vi "Write GPIO wrackpos2023.vi"(0 "Lines":tag="Dev1/port0/line0:7,Dev1/port1/line0:7,Dev1/port2/line0:7", 1 "EFC":bool, 2 "Position":i8=1 min=1 max=32, 3 "Rack Pos":i8, 6 "VTEST EN":bool=TRUE, 7 "RF EN":bool) -> ()   [LabVIEW 2023]
doc: "I. Description:\nThis example demonstrates how to write values to a digital output channel.\n\nII. Instructions for Running:\n1. Select the digital lines on the DAQ device to be written.\n2. Select a value to write.\nNote: The array control is sized for 8 lines, if using a different amount of lines, change the number of elements in the array to equal the number of lines chosen.\n\nIII. Block Diagram Steps:\n1. Create a Digital Output channel. Use one channel for all lines. You can alternatively use one channel for each line, but then use a different polymorphic version of the DAQmx Write VI.\n2. Call the Start VI to start the task.\n3. Write the digital Boolean array data in a loop until the user hits the stop button or an error occurs. This write VI writes a single sample of digital data on demand, so no timeout is necessary.\n4. Call the Clear Task VI to clear the Task.\n5. Use the popup dialog box to display an error or warning if any.\n\nIV. I/O Connections Overview:\nMake sure your signal output terminals match the Lines I/O Control. In this case wire the item to receive the signal to the first eight digital lines on your DAQ Device."
uses:
  <vilib>/Utility/error.llb/DialogType.ctl
  <vilib>/DAQmx/write.llb/DAQmx Write (Digital 1D Bool 1Chan 1Samp).vi
  <vilib>/DAQmx/create/channels.llb/DAQmx Create Channel (DO-Digital Output).vi
  <vilib>/DAQmx/miscellaneous.llb/DAQmx Fill In Error Info.vi
panel:
  # "For instructions, select Help>>Show Context Help"
  # "Channel Parameters"
  # "*The number of lines in the list must\nmatch the number of elements in\nthe array."
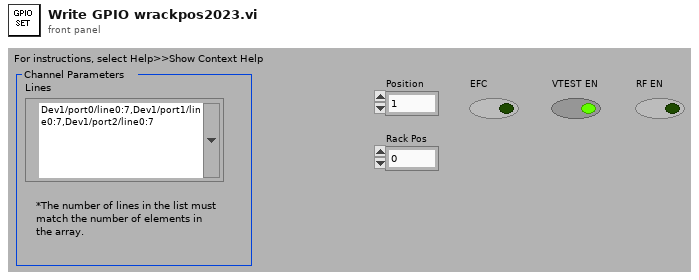
[diagram p1: front panel]
types:
  T1 = typedef "DialogType.ctl" = u16
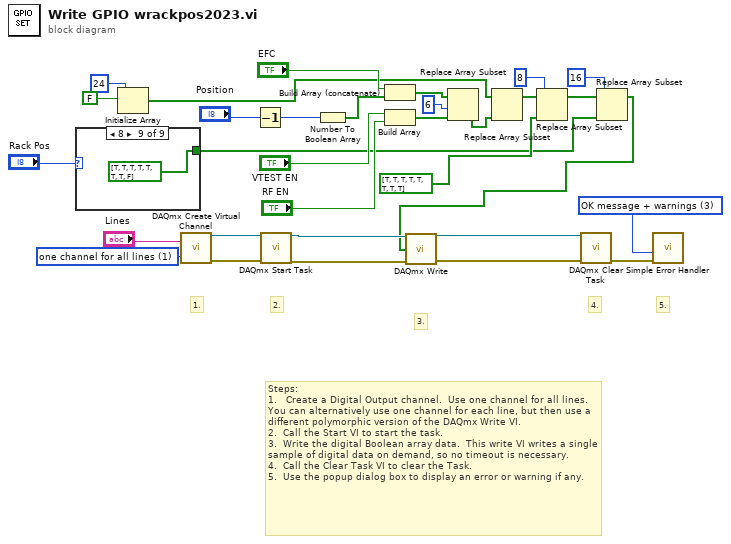
[diagram p0: block diagram]
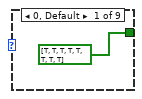
[diagram p2: hidden frame]
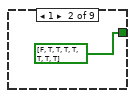
[diagram p3: hidden frame]
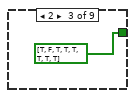
[diagram p4: hidden frame]
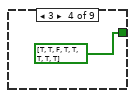
[diagram p5: hidden frame]
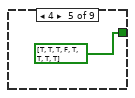
[diagram p6: hidden frame]
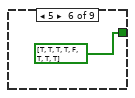
[diagram p7: hidden frame]
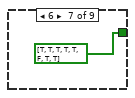
[diagram p8: hidden frame]
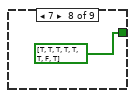
[diagram p9: hidden frame]
diagram:
  w26 = 1 items=["one channel for each line", "one channel for all lines"] ("line grouping")
  w27 = T1 3 items=["no dialog", "OK message", "continue or stop message", "OK message + warnings", "continue/stop + warnings"] ("type of dialog (OK msg:1)")
  # "3."
  # "5."
  # "Steps: \n1.   Create a Digital Output channel.  Use one channel for all lines.  You can alternatively use one channel for each line, but then use a different polymorphic version of the DAQmx Write VI.\n2.  Call the Start VI to start the task.\n3.  Write the digital Boolean array data.  This write VI writes a single sample of digital data on demand, so no timeout is necessary.\n4.  Call the Clear Task VI to clear the Task.\n5.  Use the popup dialog box to display an error or warning if any."
  # "4."
  # "2."
  # "1."
  n1 = case shown="8" "Rack Pos" {
    tunnel: [bool[] [TRUE, TRUE, TRUE, TRUE, TRUE, TRUE, TRUE, TRUE] bool[] [FALSE, TRUE, TRUE, TRUE, TRUE, TRUE, TRUE, TRUE] bool[] [TRUE, FALSE, TRUE, TRUE, TRUE, TRUE, TRUE, TRUE] bool[] [TRUE, TRUE, FALSE, TRUE, TRUE, TRUE, TRUE, TRUE] bool[] [TRUE, TRUE, TRUE, FALSE, TRUE, TRUE, TRUE, TRUE] bool[] [TRUE, TRUE, TRUE, TRUE, FALSE, TRUE, TRUE, TRUE] bool[] [TRUE, TRUE, TRUE, TRUE, TRUE, FALSE, TRUE, TRUE] bool[] [TRUE, TRUE, TRUE, TRUE, TRUE, TRUE, FALSE, TRUE] bool[] [TRUE, TRUE, TRUE, TRUE, TRUE, TRUE, TRUE, FALSE]] -> w1
    frame 0, Default {
    }
    frame 1 {
    }
    frame 2 {
    }
    frame 3 {
    }
    frame 4 {
    }
    frame 5 {
    }
    frame 6 {
    }
    frame 7 {
    }
    frame 8 {
    }
  }
  n2 = Initialize Array(FALSE, 24 ("dimension size")) -> (w10:bool[])
  n3 = call-poly <vilib>:"DAQmx Create Virtual Channel.vi"("lines"="Lines", "line grouping"=w26) -> ("task out"=w30:refnum<k21>, "error out"=w29:errorcluster)  [unwired: 12 in]
  n4 = Decrement(x="Position") -> (x-1=w14:i8)
  n5 = call <vilib>:"DAQmx Start Task.vi"("task/channels in"=w30, "error in"=w29) -> ("task out"=w25:refnum<k21>, "error out"=w24:errorcluster)  [unwired: 12 in]
  n6 = Number To Boolean Array(number=w14) -> (Boolean array=w20:bool[])
  n7 = Build Array (concatenate)("EFC", w20) -> (w15:bool[])
  n8 = Build Array("VTEST EN", "RF EN") -> (w19:bool[])
  n9 = Replace Array Subset(array=w15, new element=w19, index=6) -> (w9:bool[])
  n10 = Replace Array Subset(array=w10, new element=w9) -> (w8:bool[])  [unwired: 1 in]
  n11 = Replace Array Subset(array=w8, new element=bool[] [TRUE, TRUE, TRUE, TRUE, TRUE, TRUE, TRUE, TRUE], index=8) -> (w4:bool[])
  n12 = Replace Array Subset(array=w4, new element=w1, index=16) -> (w3:bool[])
  n13 = call-poly <vilib>:"DAQmx Write.vi"("task/channels in"=w25, "data"=w3, "error in"=w24) -> ("task out"=w23:refnum<k21>, "error out"=w22:errorcluster)  [unwired: 10 in, 1 out]
  n14 = call <vilib>:"DAQmx Clear Task.vi"("task in"=w23, "error in"=w22) -> ("error out"=w31:errorcluster)  [unwired: 13 in]
  n15 = call <vilib>:"Simple Error Handler.vi"("type of dialog (OK msg:1)"=w27, "error in (no error)"=w31) -> ()  [unwired: 3 in, 5 out]
